vi "Constants.vi"() -> ()   [LabVIEW 2015, in "Import Export Sample Custom Device Shared.lvlib"]
doc: "Use this Global VI to access the GUIDs assigned to the page resources of the Custom Device."
uses:
  Import Export Sample Custom Device Shared.lvlib
panel:
  in  "Tab Control":enum32{"GUIDS", "Constants", "Properties"}(tab)
  in  "GUIDS - Sample Channel":string="1A43963C-D3B1-4597-8095-971D7854014D"
  in  "Import Export Sample Custom Device":string="409c67da-8146-4b51-8b5e-69b89e120d34"
  in  "Sample Channel":string="Sample Channel"
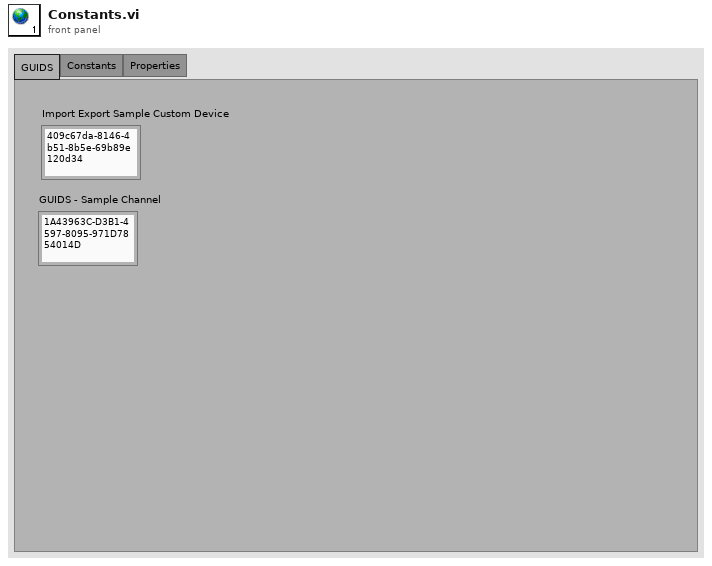
[diagram p1: front panel]
diagram:
